vi "Get Window Handle.vi"(4 "error in":errorcluster, 7 "Window Name In":string) -> (0 "error out":errorcluster, 3 "Window Handle Out":u32)   [LabVIEW 2011]
uses:
  user32.dll
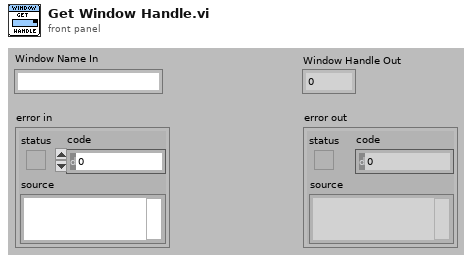
[diagram p1: front panel]
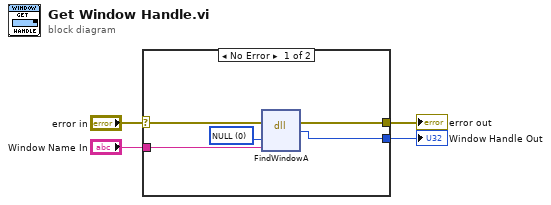
[diagram p0: block diagram]
diagram:
  n1 = case shown="No Error" "error in" {
    selector: "error in" -> [w7 w10]
    tunnel: [w6 w10] -> w2
    tunnel: [w9 _] -> w1
    tunnel: "Window Name In" -> [w8 _]
    frame No Error {
      w5 = 0 items=["NULL"]
      n2 = dll-call lib="user32.dll" fn="FindWindowA" label="FindWindow"(error in=w7, "lpszClassName"=w5, "lpszWindowName"=w8) -> (error out=w6:errorcluster, "hWnd"=w9:u32)  [unwired: 4 in, 1 out]
    }
    frame Error {
    }
  }
  "error out" <- w2
  "Window Handle Out" <- w1
